vi "Button motor control.vi"(1 "Activate Button":bool, 4 "Requested Voltage %":dbl) -> ()   [LabVIEW 2016]
uses:
  Robot Global Data.vi
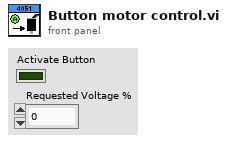
[diagram p1: front panel]
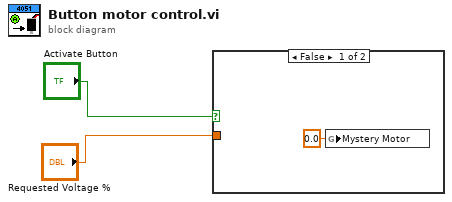
[diagram p0: block diagram]
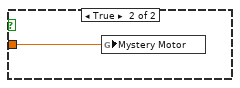
[diagram p2: hidden frame]
diagram:
  n1 = case shown="False" "Activate Button" {
    tunnel: "Requested Voltage %" -> [_ w4]
    frame False {
      n2 = global write "Robot Global Data.vi" "Mystery Motor"(0.0 ("Winch Motor")) -> ()
    }
    frame True {
      n3 = global write "Robot Global Data.vi" "Mystery Motor"(w4) -> ()
    }
  }
